vi "Global 1.vi"() -> ()   [LabVIEW 2017]
panel:
  out "우유 카메라 값":string
  out "짐빔에서 우유준비자세":string
  out "우유드는자세":string
  out "우유로 가는 자세":string
  out "우유보는자세":string
  out "술따르는자세2-2":string
  out "잭다니엘이동해야함":bool
  out "Z_부호":string
  out "Y_부호":string
  out "X_부호":string
  out "rz":dbl
  out "ry":dbl
  out "rx":dbl
  out "z":dbl
  out "y":dbl
  out "x":dbl
  out "RZ_부호":string
  out "RY_부호":string
  out "RX_부호":string
  out "지호씨가 보낸 총 좌표":string
  out "RZ_havetogo":string
  out "RY_havetogo":string
  out "RX_havetogo":string
  out "Z_havetogo":string
  out "Y_havetogo":string
  out "X_havetogo":string
  out "토닉 카메라 값":string
  out "짐빔 카메라 값":string
  out "콜라 카메라 값":string
  out "잭다니엘 카메라 값":string
  in  "TCP 스위치":bool
  in  "몇번 병을 볼것인가":string
  out "미니콜라 따르는 자세":string
  out "술잔 중간지점":string
  out "짐빔 토닉 이동 준비자세":string
  out "술 따르는 자세 2":string
  out "술잔 위로 가는 자세 2":string
  out "토닉 빼는 자세":string
  out "토닉 드는 자세":string
  out "토닉 가는자세":string
  out "토닉 보는 자세":string
  out "짐빔 들어올리는 자세":string
  out "짐빔 위치로 가는 자세":string
  out "짐빔 보는 자세":string
  out "콜라 빼는 자세":string
  out "그리퍼 닫힘":bool
  out "그리퍼 열림":bool
  out "콜라 드는 자세":string
  out "콜라로 가는자세":string
  out "콜라 보는 자세":string
  out "술 따르는 자세":string
  out "술잔 위로 가는 자세":string
  out "잭다니엘 들어올리는 자세":string
  out "잭다닐 위치로 가는 자세":string
  out "잭다니엘 보는 자세":string
  out "1자로 서는 자세":string
  out "3rd Order":bool
  out "2nd Order":bool
  out "1st Order":bool
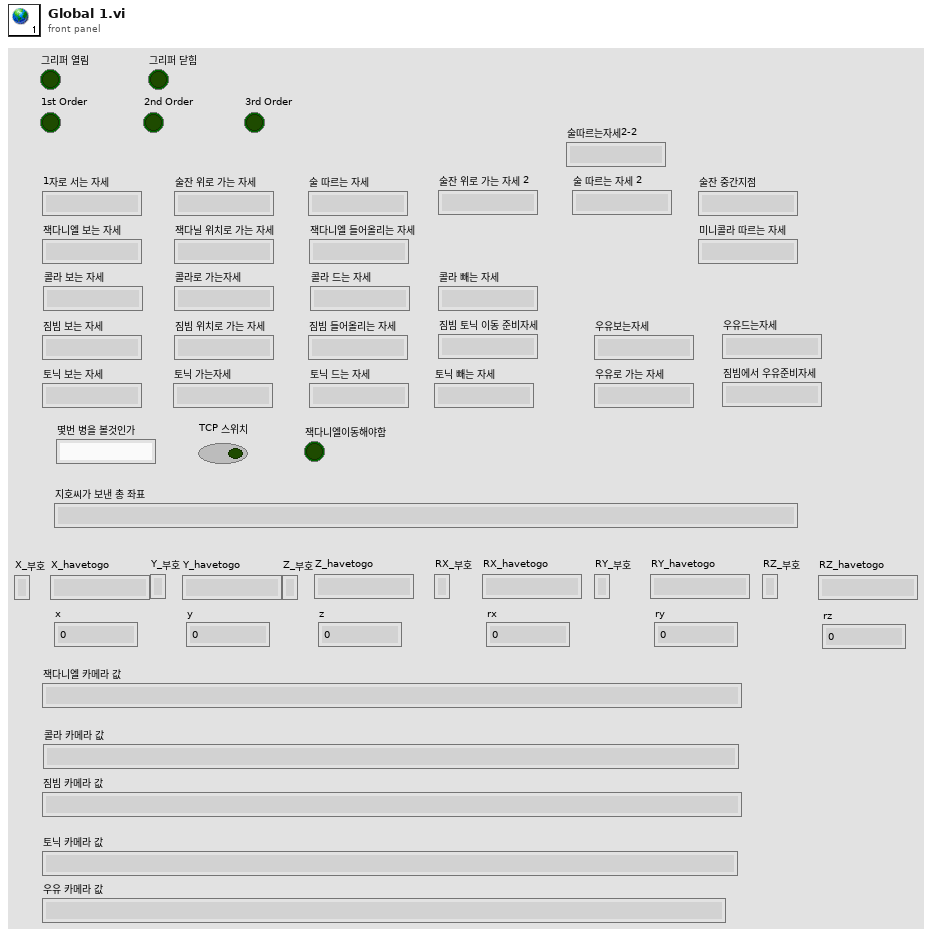
[diagram p1: front panel]
diagram:
